vi "MES_PSNR.vi"(0 "ori":dbl[][](array[numeric]), 1 "rec":dbl[][](array[numeric])) -> (3 "MSE":dbl, 4 "PSNR":dbl, 5 "SNR":dbl)   [LabVIEW 2018]
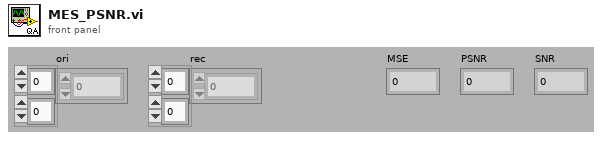
[diagram p1: front panel]
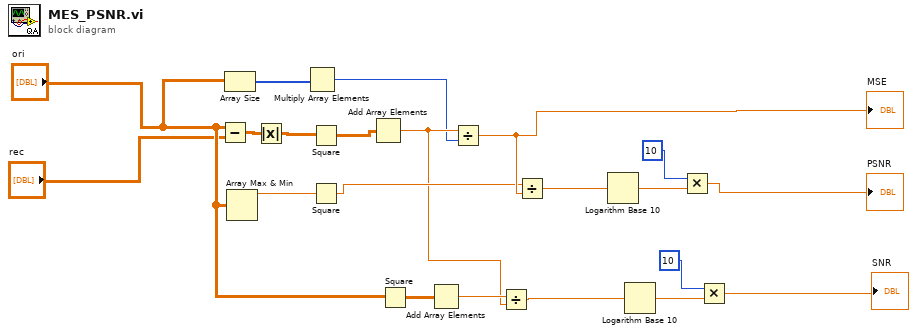
[diagram p0: block diagram]
diagram:
  n1 = Subtract(x="ori", y="rec") -> (x-y=w19:dbl[][])
  n2 = Array Size(array="ori") -> (size(s)=w16:i32[])
  n3 = Array Max & Min(array="ori") -> (max value=w15:dbl)  [unwired: 3 out]
  n4 = Absolute Value(x=w19) -> (abs(x)=w18:dbl[][])
  n5 = Multiply Array Elements(1:w16) -> (0:w7:i32)
  n6 = Square(x=w18) -> (x^2=w20:dbl[][])
  n7 = Square(x=w15) -> (x^2=w17:dbl)
  n8 = Add Array Elements(numeric array=w20) -> (sum=w8:dbl)
  n9 = Square(x="ori") -> (x^2=w10:dbl[][])
  n10 = Add Array Elements(numeric array=w10) -> (sum=w9:dbl)
  n11 = Divide(x=w8, y=w7) -> (x/y=w21:dbl)
  "MSE" <- w21
  n12 = Divide(x=w9, y=w8) -> (x/y=w4:dbl)
  n13 = Divide(x=w17, y=w21) -> (x/y=w14:dbl)
  n14 = Logarithm Base 10(1:w14) -> (0:w13:dbl)
  n15 = Logarithm Base 10(1:w4) -> (0:w5:dbl)
  n16 = Multiply(x=u8 10, y=w13) -> (x*y=→"PSNR":dbl)
  n17 = Multiply(x=u8 10, y=w5) -> (x*y=→"SNR":dbl)
